vi "Get Reference.vi"(8 "error in (no error)":errorcluster, 10 "Samples":i32, 11 "Software Lock-in in":refnum<class "Software Lock-in.lvclass">) -> (0 "error out":errorcluster, 2 "Reference":cdb[](array[numeric]), 3 "Software Lock-in out":refnum<class "Software Lock-in.lvclass">)   [LabVIEW 2016, in "Software Lock-in.lvclass"]
uses:
  Software Lock-in.lvclass
  Software Lock-in.lvclass/Software Lock-in.ctl
  <vilib>/Analysis/NI_AALBase.lvlib
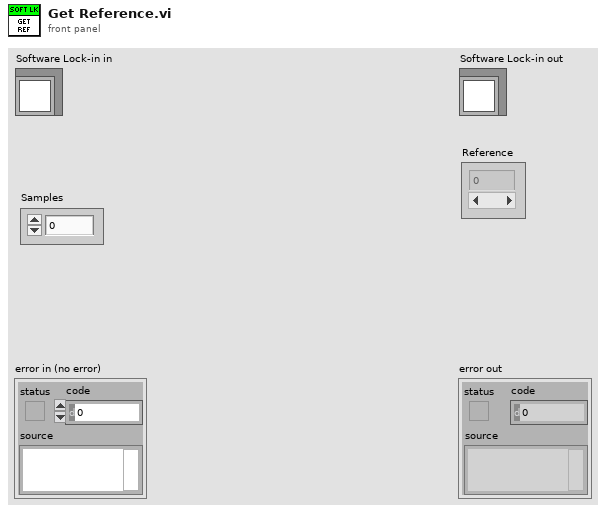
[diagram p1: front panel]
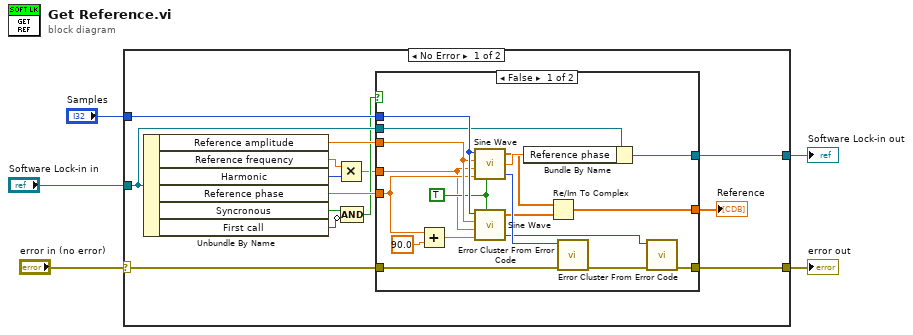
[diagram p0: block diagram]
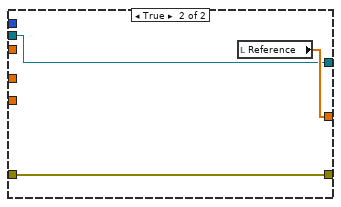
[diagram p2: hidden frame]
diagram:
  n1 = case shown="No Error" "error in (no error)" {
    selector: "error in (no error)" -> [w16 w42]
    tunnel: [w15 w42] -> w4
    tunnel: [w13 w41] -> w2
    tunnel: "Software Lock-in in" -> [w18 w41]
    tunnel: "Samples" -> [w19 _]
    frame No Error {
      n2 = Unbundle By Name(w18) -> ("Reference amplitude"=w17:dbl, "Reference frequency"=w7:dbl, "Harmonic"=w6:i32, "Reference phase"=w14:dbl, "Syncronous"=w10:bool, "First call"=w11:bool)
      n3 = Multiply(x=w7, y=w6) -> (x*y=w8:dbl)
      n4 = Compound Arithmetic op=AND(w10, invert w11) -> (w9:bool)
      n5 = case shown="False" w9 {
        tunnel: w19 -> [w35 _]
        tunnel: w18 -> [w34 w39]
        tunnel: w17 -> [w33 _]
        tunnel: w16 -> [w29 w38]
        tunnel: [w27 w38] -> w15
        tunnel: w14 -> [w26 _]
        tunnel: [w25 w39] -> w13
        tunnel: w8 -> [w23 _]
        tunnel: [w20 w40] -> w12
        frame False {
          w32 = TRUE ("reset phase")
          n6 = Add(x=w26, y=90.0) -> (x+y=w36:dbl)
          n7 = call <vilib>:"Sine Wave.vi"("samples"=w35, "amplitude"=w33, "frequency"=w23, "phase in"=w26, "reset phase"=w32) -> ("sine wave"=w22:dbl[], "phase out"=w24:dbl, "error"=w31:i32)
          n8 = call <vilib>:"Sine Wave.vi"("samples"=w35, "amplitude"=w33, "frequency"=w23, "phase in"=w36, "reset phase"=w32) -> ("sine wave"=w21:dbl[], "error"=w30:i32)  [unwired: 1 out]
          n9 = Bundle By Name(cluster=w34, "Reference phase"=w24) -> (w25:refnum<class "Software Lock-in.lvclass">)
          n10 = Re/Im To Complex(1:w21, 2:w22) -> (0:w20:cdb[])
          n11 = call <vilib>:"Error Cluster From Error Code.vi"("error in (no error)"=w29, "error code (0)"=w31) -> ("error out"=w28:errorcluster)  [unwired: 7 in]
          n12 = call <vilib>:"Error Cluster From Error Code.vi"("error in (no error)"=w28, "error code (0)"=w30) -> ("error out"=w27:errorcluster)  [unwired: 7 in]
        }
        frame True {
          n13 = local read "Reference"() -> (w40:cdb[])
        }
      }
      "Reference" <- w12
    }
    frame Error {
    }
  }
  "error out" <- w4
  "Software Lock-in out" <- w2
